vi "VibratomeGUI.vi"() -> ()   [LabVIEW 2014]
uses:
  Hardware/Table Stage/Controls/Translation Stage Cluster.ctl
  General/Controls/Translation Stage Types.ctl
  General/Controls/Translation Stage Quick Status.ctl
  General/Controls/Translation Stage Quick Controls.ctl
  General/Controls/Queue Manager Actions.ctl
  General/Controls/MessagePacket.ctl
  General/Controls/QueueNames.ctl
  <vilib>/Utility/miscctls.llb/LVPointTypeDef.ctl
  Hardware/Table Stage/Controls/Motion Translation Module Control.ctl
  General/Controls/Set Get Controls.ctl
panel:
  in  "Z STEP MOTION":enum16{"Fine", "Course", "Extra Course"}(ring)
  in  "Stop Button":bool
  in  "Slice":bool
  in  "Vibratome Controls":T1
  out "Message":string
  in  "Z Ctrl":T2
  out "Z Status":T3
  in  "Y Ctrl":T2
  out "Y Status":T3
  in  "X Ctrl":T2
  out "X Status":T3
  in  "XY STEP MOTION":enum16{"Fine", "Course", "Extra Course"}(ring)
  out "Cluster":cluster{"X":T4, "Y":T4, "Z":T4}
  in  "Exit":bool
  out "Processor Error Out":errorcluster
  out "GUI Error Out":errorcluster
  # "Vibratome Controls"
  # "Z Axis"
  # "Y Axis"
  # "X Axis"
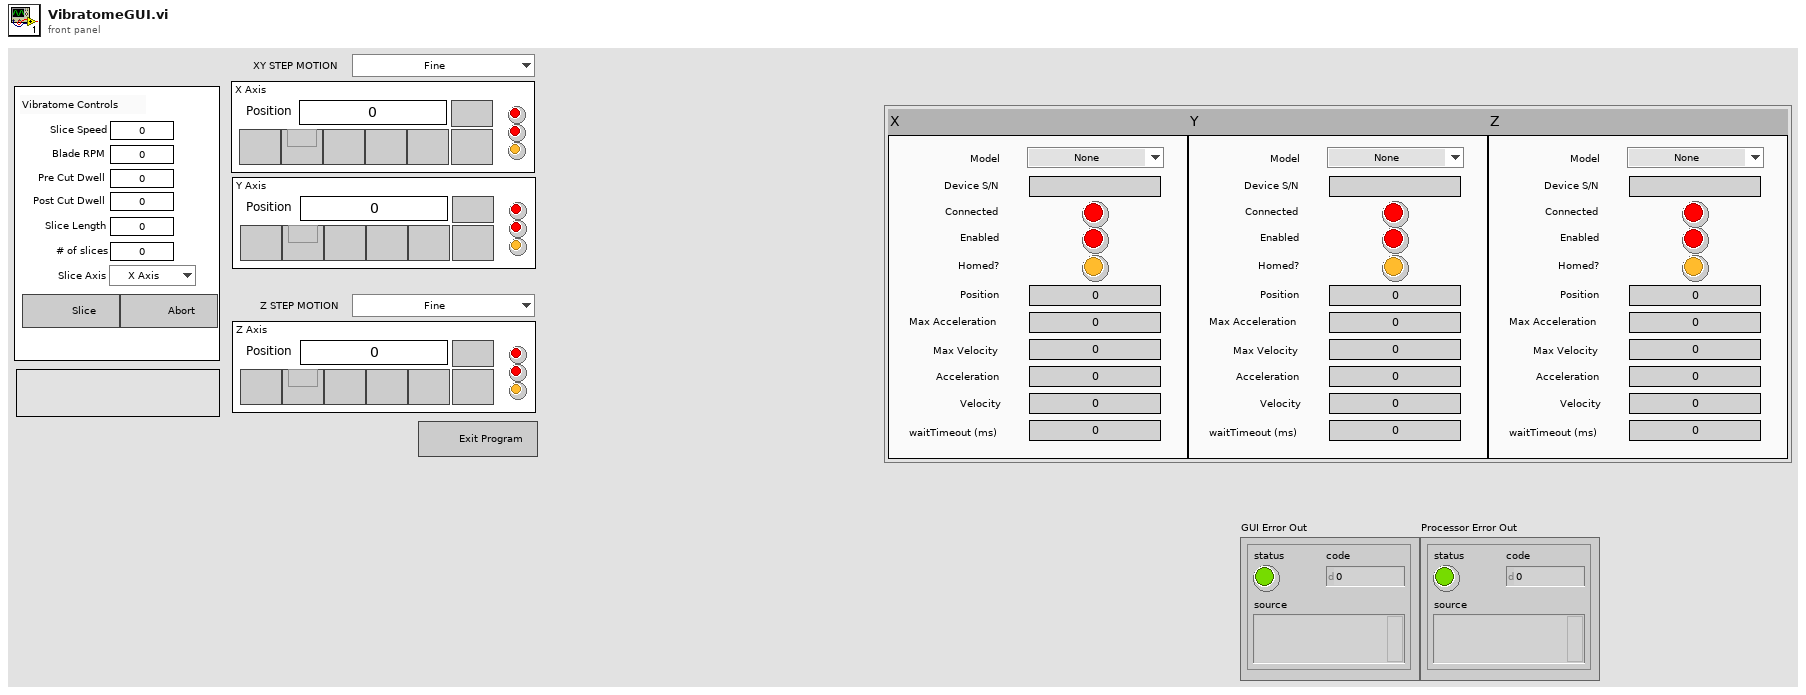
[diagram p1: front panel]
types:
  T1 = cluster{"Pre Cut Dwell":dbl, "Blade RPM":u16, "Slice Speed":dbl, "Post Cut Dwell":dbl, "Slice Length":dbl, "# of slices":dbl, "Slice Axis":enum16{"X Axis", "Y Axis", "Z Axis"}}
  T2 = typedef "Translation Stage Quick Controls.ctl" = cluster{"Position":dbl, "Next Button":bool, "Last Button":bool, "Previous Button":bool, "First Button":bool, "Home Button":bool, "Go":bool, "Settings Button":bool}
  T3 = typedef "Translation Stage Quick Status.ctl" = cluster{"Is.Enabled?":bool, "Is.Connected?":bool, "Is.Homed?":bool}
  T4 = typedef "Translation Stage Cluster.ctl" = cluster{"Position":dbl, "Is.Enabled?":bool, "Is.Connected?":bool, "Device SN":string, "AccelerationMaximum":dbl, "VelocityMaximum":dbl, "Acceleration":dbl, "Velocity":dbl, "waitTimeout (ms)":i32, "Model":T5, "Is.Homed?":bool}
  T5 = typedef "Translation Stage Types.ctl" = enum16{"None", "Thorlabs LTS", "Thorlabs MLJ"}
  T6 = typedef "MessagePacket.ctl" = cluster{"Message":string, "Parameter":variant}
  T7 = typedef "Queue Manager Actions.ctl" = enum16{"Init", "Enqueue", "Enqueue All", "Preview Queue", "Dequeue", "Get Status", "Flush Queue", "Flush All Queues", "Release All Queues", "Release Queue", "Enqueue at Opposite End"}
  T8 = typedef "QueueNames.ctl" = enum16{"Main GUI", "Main Scan Processor", "Main Display", "Main Table Stage GUI", "Main Table Stage Proc.", "Scan Engine", "Vibratome GUI", "Vibratome Processor", "Slice Engine"}
  T9 = typedef "LVPointTypeDef.ctl" = cluster{"Horizontal":i16, "Vertical":i16}
  T10 = enum16{"Set Configuration", "Get Configuration", "Enable Motor", "Disable Motor", "Get Status", "Open Session", "Close Session", "Set Limits", "Get Limits"}
  T11 = typedef "Set Get Controls.ctl" = enum16{"Set", "Get"}
  T12 = typedef "Motion Translation Module Control.ctl" = enum16{"Init", "Home", "Status", "Velocity/Accel", "Position", "Jog", "Stop", "Uninit", "Enable", "Disable"}
  T13 = cluster{"X Stage":T4, "Y Stage":T4, "Z Stage":T4}
  T14 = typedef "System Parameters.ctl" = cluster{"OCT":cluster{"Focal Length":dbl[unit]}, "Vibratome":cluster{"Z Bottom [mm]":dbl, "Pre Cut Dwell [s]":dbl, "Blade Frequency [RPM]":u16, "Slice Speed [mm/s]":dbl, "Post Cut Dwell [s]":dbl, "Ramp Time [s]":dbl, "Start X [mm]":dbl, "Start Y [mm]":dbl, "Slice Length [mm]":dbl, "Slice Axis":enum16{"X Axis", "Y Axis", "Z Axis"}, "Controller VISA Ref":refnum<visa-resource-name>}, "Table Stages":cluster{"X Stage":T4, "Y Stage":T4, "Z Stage":T4}}
  T15 = cluster{"Z Bottom [mm]":dbl, "Pre Cut Dwell [s]":dbl, "Blade Frequency [RPM]":u16, "Slice Speed [mm/s]":dbl, "Post Cut Dwell [s]":dbl, "Ramp Time [s]":dbl, "Start X [mm]":dbl, "Start Y [mm]":dbl, "Slice Length [mm]":dbl, "Slice Axis":enum16{"X Axis", "Y Axis", "Z Axis"}, "Controller VISA Ref":refnum<visa-resource-name>}
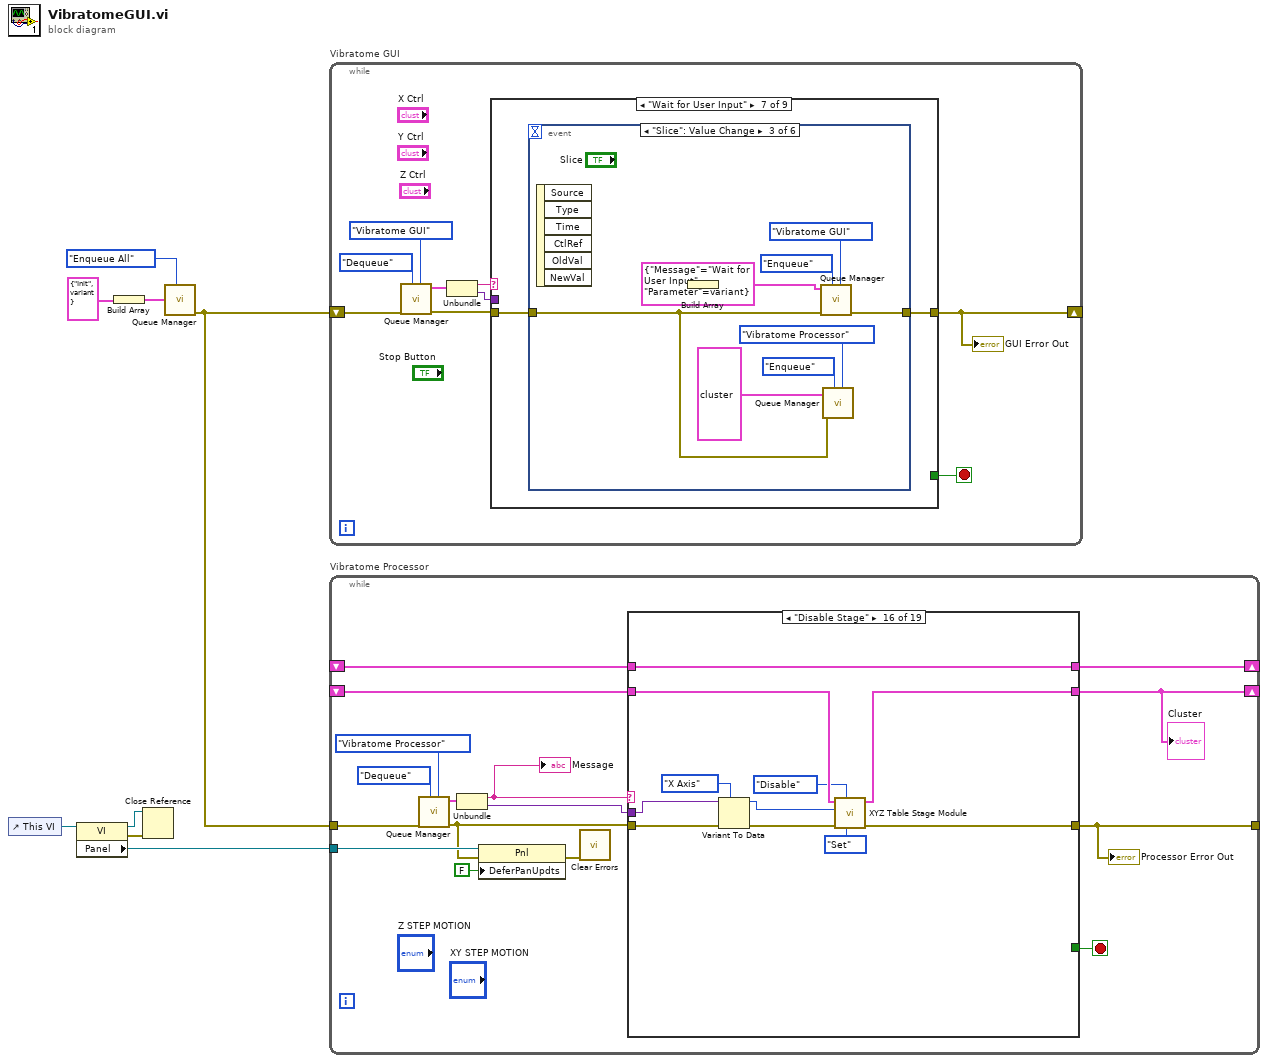
[diagram p0: block diagram]
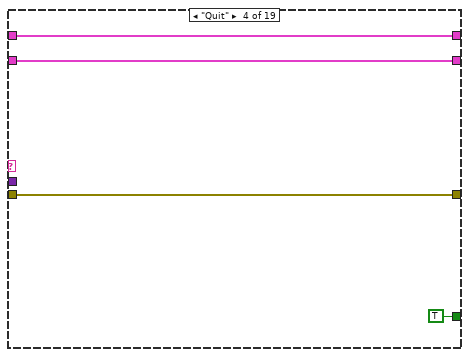
[diagram p5: hidden frame]
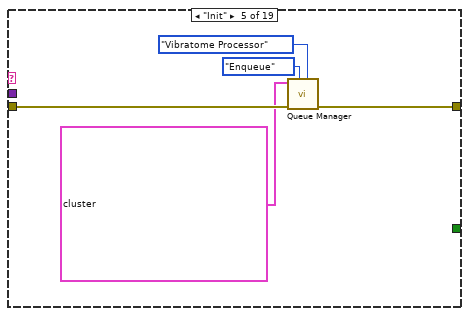
[diagram p6: hidden frame]
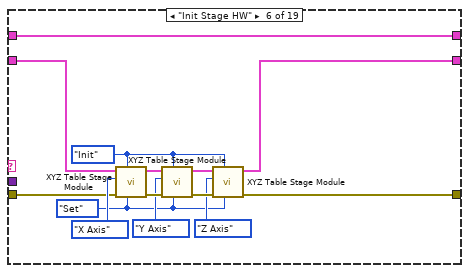
[diagram p7: hidden frame]
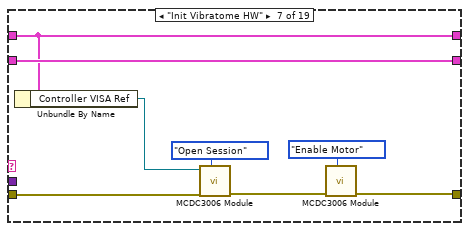
[diagram p8: hidden frame]
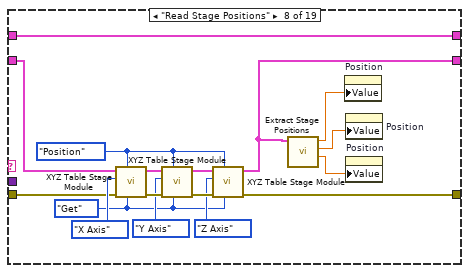
[diagram p9: hidden frame]
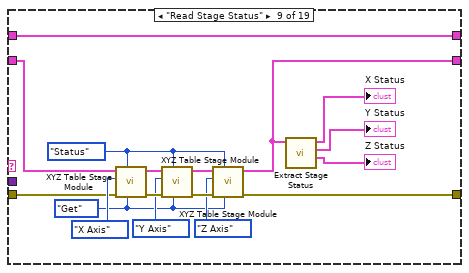
[diagram p10: hidden frame]
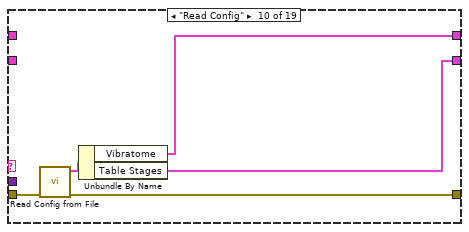
[diagram p11: hidden frame]
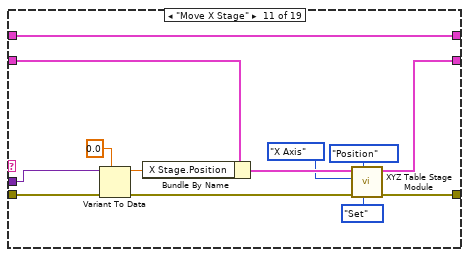
[diagram p12: hidden frame]
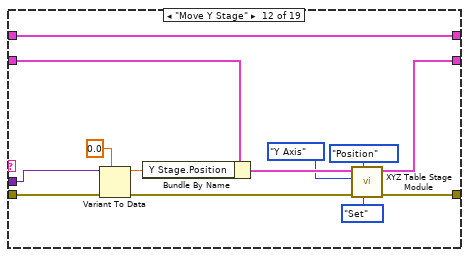
[diagram p13: hidden frame]
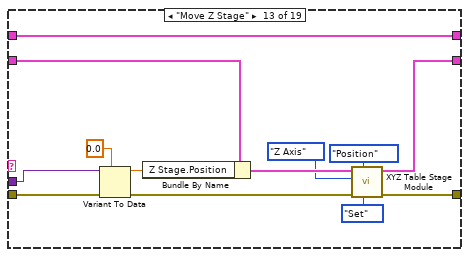
[diagram p14: hidden frame]
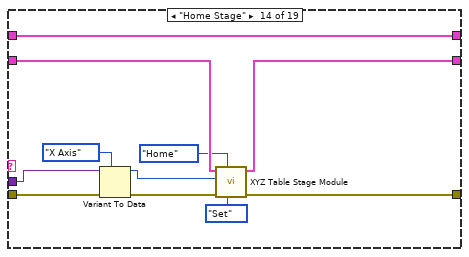
[diagram p15: hidden frame]
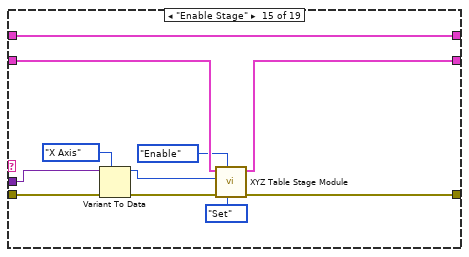
[diagram p16: hidden frame]
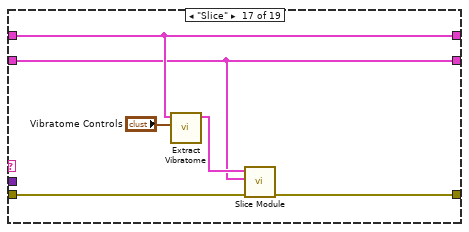
[diagram p17: hidden frame]
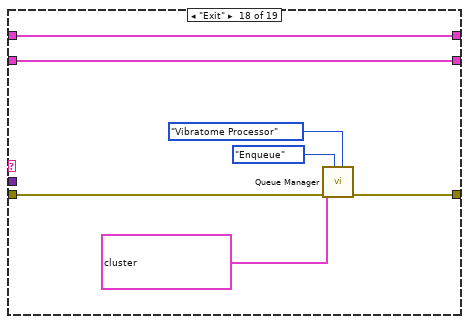
[diagram p18: hidden frame]
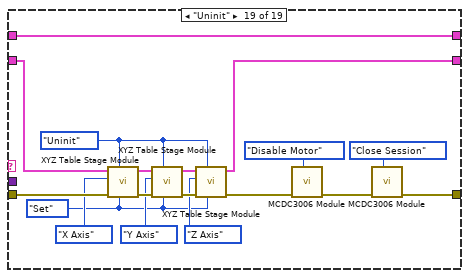
[diagram p19: hidden frame]
diagram:
  n1 = control-ref of="This VI"() -> (w4:refnum<vi>)
  n2 = property class="VI"(reference=w4) -> (reference out=w2:refnum<vi>, error out=w3:errorcluster, "Panel"=w1:refnum<vi>)  [unwired: 1 in]
  n3 = Build Array(T6 {"Message"="Init", "Parameter"=variant} ("Message Packet [In]")) -> (w6:T6[])
  n4 = Close Reference(reference=w2, error in (no error)=w3) -> ()  [unwired: 1 out]
  n5 = call "Queue Manager.vi"("Action"=Queue_Manager_Actions."Enqueue All", "Message Packet Array"=w6) -> ("Error Out"=w5:errorcluster)  [unwired: 7 in, 2 out]
  n6 = while "Vibratome GUI" {
    shift-right: [w17] -> _
    shift-left: w5 -> [w15]
    stop <- w10 stop-if-true
    n7 = call "Queue Manager.vi"("Queue Name"=QueueNames."Vibratome GUI", "Action"=Queue_Manager_Actions."Dequeue", "Error In"=w15) -> ("Error Out"=w14:errorcluster, "Message Packet [Out]"=w13:T6)  [unwired: 6 in, 1 out]
    n8 = Unbundle(w13) -> ("Message"=w12:string, "Parameter"=w11:variant)
    n9 = case shown="\"Wait for User Input\"" w12 {
      tunnel: w14 -> [w18 w19 w24 w25 w26 w27 w29 w90 w103]
      tunnel: [w18 w20 w24 w25 w26 w27 w28 w91 w103] -> w17
      tunnel: w11 -> [_ _ _ _ _ _ _ _ _]
      tunnel: [_ _ _ _ _ _ _ _ TRUE] -> w10
      frame "Unknown", Default {
      }
      frame "Init" {
        n10 = call "Queue Manager.vi"("Queue Name"=QueueNames."Vibratome GUI", "Action"=Queue_Manager_Actions."Enqueue", "Error In"=w19, "Message Packet Array"=T6[] [{"Message"="Init Variables", "Parameter"=variant}, {"Message"="Set Front Panel", "Parameter"=variant}, {"Message"="Load User Settings", "Parameter"=variant}, {"Message"="Configure Hardware", "Parameter"=variant}, {"Message"="Wait for Complete", "Parameter"=variant}, {"Message"="Wait for User Input", "Parameter"=variant}]) -> ("Error Out"=w20:errorcluster)  [unwired: 5 in, 2 out]
      }
      frame "Init Variables" {
      }
      frame "Load User Settings" {
      }
      frame "Configure Hardware" {
      }
      frame "Wait for Complete" {
      }
      frame "Wait for User Input" {
        n11 = event shown="[2] \"Slice\": Value Change" {
          selector: _ -> [_ _ _ _ _ _]
          dyn-events: _ -> [_ _ _ _ _ _]
          timeout: _ -> [_ _ _ _ _ _]
          tunnel: w29 -> [w30 w34 w37 w59 w74 w89]
          tunnel: [w30 w33 w42 w46 w61 w76] -> w28
          event Timeout {
            n12 = event-data() -> ()  [unwired: 1 in, 3 out]
          }
          event Panel Close; Application Instance Close; "Exit": Value Change {
            n13 = event-data() -> ()  [unwired: 1 in, 3 out]
            n14 = Build Array(T6 {"Message"="Exit", "Parameter"=variant} ("Message Packet [In]")) -> (w31:T6[])
            n15 = call "Queue Manager.vi"("Action"=Queue_Manager_Actions."Enqueue All", "Error In"=w34, "Message Packet Array"=w31) -> ("Error Out"=w33:errorcluster)  [unwired: 6 in, 2 out]
          }
          event "Slice": Value Change {
            n16 = event-data() -> ()  [unwired: 1 in, 6 out]
            n17 = Build Array(T6 {"Message"="Wait for User Input", "Parameter"=variant} ("Message Packet [In]")) -> (w40:T6[])
            n18 = call "Queue Manager.vi"("Queue Name"=QueueNames."Vibratome GUI", "Action"=Queue_Manager_Actions."Enqueue", "Error In"=w37, "Message Packet Array"=w40) -> ("Error Out"=w42:errorcluster)  [unwired: 5 in, 2 out]
            n19 = call "Queue Manager.vi"("Queue Name"=QueueNames."Vibratome Processor", "Action"=Queue_Manager_Actions."Enqueue", "Error In"=w37, "Message Packet Array"=T6[] [{"Message"="Slice", "Parameter"=variant}, {"Message"="Finished", "Parameter"=variant}]) -> ()  [unwired: 5 in, 3 out]
          }
          event Value Change {
            n20 = event-data() -> ()  [unwired: 1 in, 1 out]
            n21 = property on="Position" class="DigNum (strict)"(error in=w59) -> (error out=w56:errorcluster, "Value"=w54:dbl)  [unwired: 1 in, 1 out]
            n22 = Bundle By Name(cluster=T6 {"Message"="Move X Stage", "Parameter"=variant} ("Message Packet [In]"), "Parameter"=w54) -> (w53:T6)
            n23 = Build Array(w53, T6 {"Message"="Finished", "Parameter"=variant} ("Message Packet [In]")) -> (w52:T6[])
            n24 = call "Queue Manager.vi"("Queue Name"=QueueNames."Vibratome Processor", "Action"=Queue_Manager_Actions."Enqueue", "Error In"=w56, "Message Packet Array"=w52) -> ("Error Out"=w47:errorcluster)  [unwired: 5 in, 2 out]
            n25 = Build Array(T6 {"Message"="Wait for User Input", "Parameter"=variant} ("Message Packet [In]")) -> (w48:T6[])
            n26 = call "Queue Manager.vi"("Queue Name"=QueueNames."Vibratome GUI", "Action"=Queue_Manager_Actions."Enqueue", "Error In"=w47, "Message Packet Array"=w48) -> ("Error Out"=w46:errorcluster)  [unwired: 5 in, 2 out]
          }
          event Value Change {
            n27 = event-data() -> ()  [unwired: 1 in, 1 out]
            n28 = property on="Position" class="DigNum (strict)"(error in=w74) -> (error out=w71:errorcluster, "Value"=w69:dbl)  [unwired: 1 in, 1 out]
            n29 = Bundle By Name(cluster=T6 {"Message"="Move Y Stage", "Parameter"=variant} ("Message Packet [In]"), "Parameter"=w69) -> (w68:T6)
            n30 = Build Array(w68, T6 {"Message"="Finished", "Parameter"=variant} ("Message Packet [In]")) -> (w67:T6[])
            n31 = call "Queue Manager.vi"("Queue Name"=QueueNames."Vibratome Processor", "Action"=Queue_Manager_Actions."Enqueue", "Error In"=w71, "Message Packet Array"=w67) -> ("Error Out"=w62:errorcluster)  [unwired: 5 in, 2 out]
            n32 = Build Array(T6 {"Message"="Wait for User Input", "Parameter"=variant} ("Message Packet [In]")) -> (w63:T6[])
            n33 = call "Queue Manager.vi"("Queue Name"=QueueNames."Vibratome GUI", "Action"=Queue_Manager_Actions."Enqueue", "Error In"=w62, "Message Packet Array"=w63) -> ("Error Out"=w61:errorcluster)  [unwired: 5 in, 2 out]
          }
          event Value Change {
            n34 = event-data() -> ()  [unwired: 1 in, 1 out]
            n35 = property on="Position" class="DigNum (strict)"(error in=w89) -> (error out=w86:errorcluster, "Value"=w84:dbl)  [unwired: 1 in, 1 out]
            n36 = Bundle By Name(cluster=T6 {"Message"="Move Z Stage", "Parameter"=variant} ("Message Packet [In]"), "Parameter"=w84) -> (w83:T6)
            n37 = Build Array(w83, T6 {"Message"="Finished", "Parameter"=variant} ("Message Packet [In]")) -> (w82:T6[])
            n38 = call "Queue Manager.vi"("Queue Name"=QueueNames."Vibratome Processor", "Action"=Queue_Manager_Actions."Enqueue", "Error In"=w86, "Message Packet Array"=w82) -> ("Error Out"=w77:errorcluster)  [unwired: 5 in, 2 out]
            n39 = Build Array(T6 {"Message"="Wait for User Input", "Parameter"=variant} ("Message Packet [In]")) -> (w78:T6[])
            n40 = call "Queue Manager.vi"("Queue Name"=QueueNames."Vibratome GUI", "Action"=Queue_Manager_Actions."Enqueue", "Error In"=w77, "Message Packet Array"=w78) -> ("Error Out"=w76:errorcluster)  [unwired: 5 in, 2 out]
          }
        }
      }
      frame "Set Front Panel" {
        n41 = control-ref of="This VI"() -> (w92:refnum<vi>)
        n42 = property class="VI"(reference=w92, error in=w90) -> (error out=w94:errorcluster, "Panel"=w97:refnum<vi>)  [unwired: 1 out]
        n43 = property class="Pnl"(reference=w97, error in=w94) -> (error out=w95:errorcluster, "Panes[]"=w96:refnum<vi>[])  [unwired: 1 out]
        n44 = for {
          tunnel: w96 -> [w101] mode=indexing
          tunnel: w95 -> [w99]
          tunnel: [w98] -> w93 mode=indexing
          n45 = property class="Pane"(reference=w101, error in=w99, "Origin"=T9 {"Horizontal"=0, "Vertical"=0}) -> (error out=w98:errorcluster)  [unwired: 1 out]
        }
        n46 = Merge Errors(w93) -> (w91:errorcluster)
      }
      frame "Exit" {
      }
    }
    "GUI Error Out" <- w17
  }
  n47 = while "Vibratome Processor" {
    tunnel: w5 -> [w117]
    tunnel: [w119] -> _
    shift-right: [w108] -> _
    shift-left: _ -> [w111]
    shift-right: [w110] -> _
    shift-left: _ -> [w109]
    tunnel: w1 -> [w107]
    stop <- w113 stop-if-true
    n48 = call "Queue Manager.vi"("Queue Name"=QueueNames."Vibratome Processor", "Action"=Queue_Manager_Actions."Dequeue", "Error In"=w117) -> ("Error Out"=w105:errorcluster, "Message Packet [Out]"=w116:T6)  [unwired: 6 in, 1 out]
    n49 = Unbundle(w116) -> ("Message"=w115:string, "Parameter"=w114:variant)
    "Message" <- w115
    n50 = property class="Pnl"(reference=w107, error in=w105, "DeferPanUpdts"=FALSE ("Defer Panel Updates")) -> (error out=w104:errorcluster)  [unwired: 1 out]
    n51 = call <vilib>:"Clear Errors.vi"("error in (no error)"=w104) -> ()  [unwired: 5 in, 2 out]
    n52 = case shown="\"Disable Stage\"" w115 {
      tunnel: w105 -> [w122 w125 w126 w130 w137 w141 w157 w166 w183 w198 w211 w224 w237 w248 w259 w270 w275 w281 w301]
      tunnel: [w122 w125 w126 w130 w136 w149 w153 w174 w191 w195 w210 w223 w236 w247 w258 w269 w274 w280 w285] -> w119
      tunnel: w114 -> [_ _ _ _ _ _ _ _ _ _ w208 w221 w234 w245 w256 w267 _ _ _]
      tunnel: [_ _ _ TRUE _ _ _ _ _ _ _ _ _ _ _ _ _ _ _] -> w113
      tunnel: [w121 w124 w128 w132 _ w138 w159 w160 w181 w196 w207 w220 w233 w241 w252 w263 w272 w282 w294] -> w108
      tunnel: w111 -> [w121 w124 w128 w132 _ w140 w159 w165 w182 _ w203 w216 w229 w242 w253 w264 w272 w282 w297]
      tunnel: [w120 w123 w127 w131 _ w139 w155 w164 w177 w194 w199 w212 w225 w238 w249 w260 w276 w283 w288] -> w110
      tunnel: w109 -> [w120 w123 w127 w131 _ w139 w155 w164 w177 _ w199 w212 w225 w238 w249 w260 w276 w283 w288]
      frame "Unknown", Default {
      }
      frame "Finished Init" {
      }
      frame "Finished" {
      }
      frame "Quit" {
      }
      frame "Init" {
        n53 = call "Queue Manager.vi"("Queue Name"=QueueNames."Vibratome Processor", "Action"=Queue_Manager_Actions."Enqueue", "Error In"=w137, "Message Packet Array"=T6[] [{"Message"="Read Config", "Parameter"=variant}, {"Message"="Init Stage HW", "Parameter"=variant}, {"Message"="Read Stage Status", "Parameter"=variant}, {"Message"="Read Stage Positions", "Parameter"=variant}, {"Message"="Init Vibratome HW", "Parameter"=variant}, {"Message"="Finished Init", "Parameter"=variant}]) -> ("Error Out"=w136:errorcluster)  [unwired: 5 in, 2 out]
      }
      frame "Init Stage HW" {
        w142 = Set_Get_Controls."Set" ("Set/Get")
        w148 = Motion_Translation_Module_Control."Init" ("Action")
        n54 = call "XYZ Table Stage Module.vi"("Set/Get"=w142, "Action"=w148, "Error In"=w141, "Axis"=enum16{"X Axis", "Y Axis", "Z Axis"}."X Axis", "Table Stages"=w140) -> ("Error Out"=w151:errorcluster, "Table Stages Out"=w147:T13)  [unwired: 5 in]
        n55 = call "XYZ Table Stage Module.vi"("Set/Get"=w142, "Action"=w148, "Error In"=w151, "Axis"=enum16{"X Axis", "Y Axis", "Z Axis"}."Y Axis", "Table Stages"=w147) -> ("Error Out"=w150:errorcluster, "Table Stages Out"=w146:T13)  [unwired: 5 in]
        n56 = call "XYZ Table Stage Module.vi"("Set/Get"=w142, "Action"=w148, "Error In"=w150, "Axis"=enum16{"X Axis", "Y Axis", "Z Axis"}."Z Axis", "Table Stages"=w146) -> ("Error Out"=w149:errorcluster, "Table Stages Out"=w138:T13)  [unwired: 5 in]
      }
      frame "Init Vibratome HW" {
        n57 = Unbundle By Name(w155) -> ("Controller VISA Ref"=w154:refnum<visa-resource-name>)
        n58 = call "MCDC3006 Module.vi"("Actions"=T10."Open Session", "Error In"=w157, "VISA resource name"=w154) -> ("Error Out"=w156:errorcluster)  [unwired: 4 in, 4 out]
        n59 = call "MCDC3006 Module.vi"("Actions"=T10."Enable Motor", "Error In"=w156) -> ("Error Out"=w153:errorcluster)  [unwired: 5 in, 4 out]
      }
      frame "Read Stage Positions" {
        w167 = Set_Get_Controls."Get" ("Set/Get")
        w173 = Motion_Translation_Module_Control."Position" ("Action")
        n60 = call "XYZ Table Stage Module.vi"("Set/Get"=w167, "Action"=w173, "Error In"=w166, "Axis"=enum16{"X Axis", "Y Axis", "Z Axis"}."X Axis", "Table Stages"=w165) -> ("Error Out"=w176:errorcluster, "Table Stages Out"=w172:T13)  [unwired: 5 in]
        n61 = call "XYZ Table Stage Module.vi"("Set/Get"=w167, "Action"=w173, "Error In"=w176, "Axis"=enum16{"X Axis", "Y Axis", "Z Axis"}."Y Axis", "Table Stages"=w172) -> ("Error Out"=w175:errorcluster, "Table Stages Out"=w171:T13)  [unwired: 5 in]
        n62 = call "XYZ Table Stage Module.vi"("Set/Get"=w167, "Action"=w173, "Error In"=w175, "Axis"=enum16{"X Axis", "Y Axis", "Z Axis"}."Z Axis", "Table Stages"=w171) -> ("Error Out"=w174:errorcluster, "Table Stages Out"=w160:T13)  [unwired: 5 in]
        n63 = call "Extract Stage Positions.vi"("Table Stages"=w160) -> ("Z Stage.Position"=w161:dbl, "Y Stage.Position"=w162:dbl, "X Stage.Position"=w163:dbl)  [unwired: 8 in]
        n64 = property on="Position" class="DigNum (strict)"("Value"=w163) -> ()  [unwired: 2 in, 2 out]
        n65 = property on="Position" class="DigNum (strict)"("Value"=w162) -> ()  [unwired: 2 in, 2 out]
        n66 = property on="Position" class="DigNum (strict)"("Value"=w161) -> ()  [unwired: 2 in, 2 out]
      }
      frame "Read Stage Status" {
        w184 = Set_Get_Controls."Get" ("Set/Get")
        w190 = Motion_Translation_Module_Control."Status" ("Action")
        n67 = call "XYZ Table Stage Module.vi"("Set/Get"=w184, "Action"=w190, "Error In"=w183, "Axis"=enum16{"X Axis", "Y Axis", "Z Axis"}."X Axis", "Table Stages"=w182) -> ("Error Out"=w193:errorcluster, "Table Stages Out"=w189:T13)  [unwired: 5 in]
        n68 = call "XYZ Table Stage Module.vi"("Set/Get"=w184, "Action"=w190, "Error In"=w193, "Axis"=enum16{"X Axis", "Y Axis", "Z Axis"}."Y Axis", "Table Stages"=w189) -> ("Error Out"=w192:errorcluster, "Table Stages Out"=w188:T13)  [unwired: 5 in]
        n69 = call "XYZ Table Stage Module.vi"("Set/Get"=w184, "Action"=w190, "Error In"=w192, "Axis"=enum16{"X Axis", "Y Axis", "Z Axis"}."Z Axis", "Table Stages"=w188) -> ("Error Out"=w191:errorcluster, "Table Stages Out"=w181:T13)  [unwired: 5 in]
        n70 = call "Extract Stage Status.vi"("Table Stages"=w181) -> ("Z Stage"=→"Z Status":T3, "Y Stage"=→"Y Status":T3, "X Stage"=→"X Status":T3)  [unwired: 8 in]
      }
      frame "Read Config" {
        n71 = call "Read Config from File.vi"("error in (no error)"=w198) -> ("error out"=w195:errorcluster, "System Parameters"=w197:T14)  [unwired: 9 in]
        n72 = Unbundle By Name(w197) -> ("Vibratome"=w194:T15, "Table Stages"=w196:T13)
      }
      frame "Move X Stage" {
        n73 = Variant To Data(error in=w211, type=0.0 ("Value"), Variant=w208) -> (data=w202:dbl, error out=w209:errorcluster)
        n74 = Bundle By Name(cluster=w203, "X Stage.Position"=w202) -> (w201:T13)
        n75 = call "XYZ Table Stage Module.vi"("Set/Get"=Set_Get_Controls."Set", "Action"=Motion_Translation_Module_Control."Position", "Error In"=w209, "Axis"=enum16{"X Axis", "Y Axis", "Z Axis"}."X Axis", "Table Stages"=w201) -> ("Error Out"=w210:errorcluster, "Table Stages Out"=w207:T13)  [unwired: 5 in]
      }
      frame "Move Y Stage" {
        n76 = Variant To Data(error in=w224, type=0.0 ("Value"), Variant=w221) -> (data=w215:dbl, error out=w222:errorcluster)
        n77 = Bundle By Name(cluster=w216, "Y Stage.Position"=w215) -> (w214:T13)
        n78 = call "XYZ Table Stage Module.vi"("Set/Get"=Set_Get_Controls."Set", "Action"=Motion_Translation_Module_Control."Position", "Error In"=w222, "Axis"=enum16{"X Axis", "Y Axis", "Z Axis"}."Y Axis", "Table Stages"=w214) -> ("Error Out"=w223:errorcluster, "Table Stages Out"=w220:T13)  [unwired: 5 in]
      }
      frame "Move Z Stage" {
        n79 = Variant To Data(error in=w237, type=0.0 ("Value"), Variant=w234) -> (data=w228:dbl, error out=w235:errorcluster)
        n80 = Bundle By Name(cluster=w229, "Z Stage.Position"=w228) -> (w227:T13)
        n81 = call "XYZ Table Stage Module.vi"("Set/Get"=Set_Get_Controls."Set", "Action"=Motion_Translation_Module_Control."Position", "Error In"=w235, "Axis"=enum16{"X Axis", "Y Axis", "Z Axis"}."Z Axis", "Table Stages"=w227) -> ("Error Out"=w236:errorcluster, "Table Stages Out"=w233:T13)  [unwired: 5 in]
      }
      frame "Home Stage" {
        n82 = Variant To Data(error in=w248, type=enum16{"X Axis", "Y Axis", "Z Axis"}."X Axis" ("Axis"), Variant=w245) -> (data=w243:enum16{"X Axis", "Y Axis", "Z Axis"}, error out=w246:errorcluster)
        n83 = call "XYZ Table Stage Module.vi"("Set/Get"=Set_Get_Controls."Set", "Action"=Motion_Translation_Module_Control."Home", "Error In"=w246, "Axis"=w243, "Table Stages"=w242) -> ("Error Out"=w247:errorcluster, "Table Stages Out"=w241:T13)  [unwired: 5 in]
      }
      frame "Enable Stage" {
        n84 = Variant To Data(error in=w259, type=enum16{"X Axis", "Y Axis", "Z Axis"}."X Axis" ("Axis"), Variant=w256) -> (data=w254:enum16{"X Axis", "Y Axis", "Z Axis"}, error out=w257:errorcluster)
        n85 = call "XYZ Table Stage Module.vi"("Set/Get"=Set_Get_Controls."Set", "Action"=Motion_Translation_Module_Control."Enable", "Error In"=w257, "Axis"=w254, "Table Stages"=w253) -> ("Error Out"=w258:errorcluster, "Table Stages Out"=w252:T13)  [unwired: 5 in]
      }
      frame "Disable Stage" {
        n86 = Variant To Data(error in=w270, type=enum16{"X Axis", "Y Axis", "Z Axis"}."X Axis" ("Axis"), Variant=w267) -> (data=w265:enum16{"X Axis", "Y Axis", "Z Axis"}, error out=w268:errorcluster)
        n87 = call "XYZ Table Stage Module.vi"("Set/Get"=Set_Get_Controls."Set", "Action"=Motion_Translation_Module_Control."Disable", "Error In"=w268, "Axis"=w265, "Table Stages"=w264) -> ("Error Out"=w269:errorcluster, "Table Stages Out"=w263:T13)  [unwired: 5 in]
      }
      frame "Slice" {
        n88 = call "Extract Vibratome.vi"("Vibratome Controls"="Vibratome Controls", "Vibratome"=w276) -> ("Vibratome Out"=w273:T15)  [unwired: 9 in]
        n89 = call "Slice Module.vi"("Error In"=w275, "Table Stages"=w272, "Vibratome"=w273) -> ("Error Out"=w274:errorcluster)  [unwired: 6 in, 2 out]
      }
      frame "Exit" {
        n90 = call "Queue Manager.vi"("Queue Name"=QueueNames."Vibratome Processor", "Action"=Queue_Manager_Actions."Enqueue", "Error In"=w281, "Message Packet Array"=T6[] [{"Message"="Uninit", "Parameter"=variant}, {"Message"="Quit", "Parameter"=variant}]) -> ("Error Out"=w280:errorcluster)  [unwired: 5 in, 2 out]
      }
      frame "Uninit" {
        w289 = Set_Get_Controls."Set" ("Set/Get")
        w293 = Motion_Translation_Module_Control."Uninit" ("Action")
        n91 = call "XYZ Table Stage Module.vi"("Set/Get"=w289, "Action"=w293, "Error In"=w301, "Axis"=enum16{"X Axis", "Y Axis", "Z Axis"}."X Axis", "Table Stages"=w297) -> ("Error Out"=w299:errorcluster, "Table Stages Out"=w296:T13)  [unwired: 5 in]
        n92 = call "XYZ Table Stage Module.vi"("Set/Get"=w289, "Action"=w293, "Error In"=w299, "Axis"=enum16{"X Axis", "Y Axis", "Z Axis"}."Y Axis", "Table Stages"=w296) -> ("Error Out"=w300:errorcluster, "Table Stages Out"=w295:T13)  [unwired: 5 in]
        n93 = call "XYZ Table Stage Module.vi"("Set/Get"=w289, "Action"=w293, "Error In"=w300, "Axis"=enum16{"X Axis", "Y Axis", "Z Axis"}."Z Axis", "Table Stages"=w295) -> ("Error Out"=w298:errorcluster, "Table Stages Out"=w294:T13)  [unwired: 5 in]
        n94 = call "MCDC3006 Module.vi"("Actions"=T10."Disable Motor", "Error In"=w298) -> ("Error Out"=w287:errorcluster)  [unwired: 5 in, 4 out]
        n95 = call "MCDC3006 Module.vi"("Actions"=T10."Close Session", "Error In"=w287) -> ("Error Out"=w285:errorcluster)  [unwired: 5 in, 4 out]
      }
    }
    "Processor Error Out" <- w119
    "Cluster" <- w108
  }
